vi "XML setApiResponse.vi"(11 "PIM API Response":T1={"#attributes"={"xmlns"="http://www.summitekinstruments.com", "xmlns:xsi"="http://www.w3.org/2001/XMLSchema-instance", "xsi:schemaLocation"="http://www.summitekinstruments.com PIMXMLSchema.xsd"}, "Responses"={"#attributes"={"Legacy"=FALSE}, "Response"=[]}}) -> (3 "Formatted XML":string, 5 "Time to Translate":u32)   [LabVIEW 2011]
uses:
  Controls/PIM.API.RESPONSE.ctl
  Controls/PIM.API.Response.Collection.ctl
  Controls/PIM.API.Response.Unique.ctl
  Controls/PIM.API.Response.Samples.ctl
  WebEngine/LIB/MODULES/TR Module/Triasx.LIB/iQA Sweep Behavior.ctl
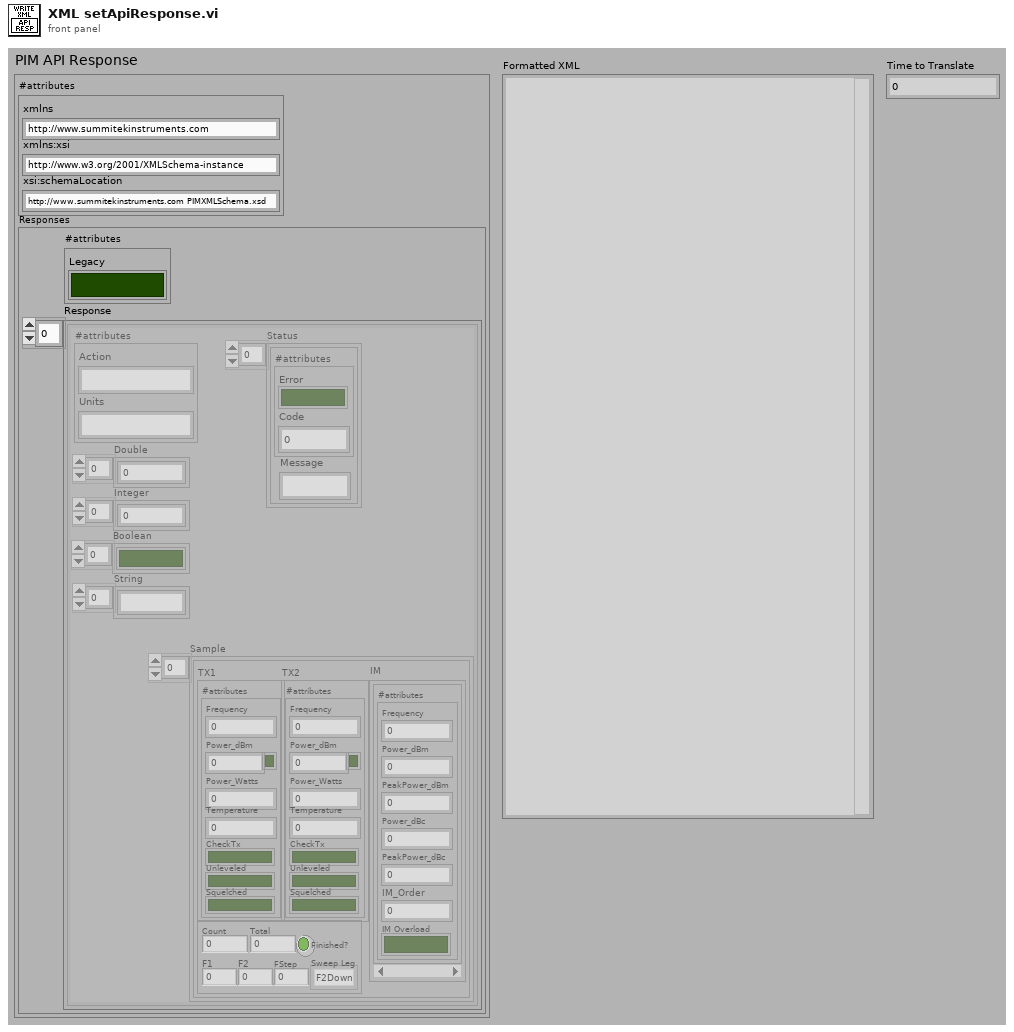
[diagram p1: front panel]
types:
  T1 = typedef "PIM.API.RESPONSE.ctl" = cluster{"#attributes":cluster{"xmlns":string, "xmlns:xsi":string, "xsi:schemaLocation":string}, "Responses":T2}
  T2 = typedef "PIM.API.Response.Collection.ctl" = cluster{"#attributes":cluster{"Legacy":bool}, "Response":T3[]}
  T3 = typedef "PIM.API.Response.Unique.ctl" = cluster{"#attributes":cluster{"Action":string, "Units":string}, "Double":dbl[], "Integer":i32[], "Boolean":bool[], "String":string[], "Sample":T4[], "Status":cluster{"#attributes":cluster{"Error":bool, "Code":i32}, "Message":string}[]}
  T4 = typedef "PIM.API.Response.Samples.ctl" = cluster{"TX1":cluster{"#attributes":cluster{"Frequency":dbl, "Power_dBm":dbl, "Power_Watts":dbl, "CheckTx":bool, "Unleveled":bool, "Squelched":bool, "Temperature":dbl, "ToneOn":bool}}, "TX2":cluster{"#attributes":cluster{"Frequency":dbl, "Power_dBm":dbl, "Power_Watts":dbl, "CheckTx":bool, "Unleveled":bool, "Squelched":bool, "Temperature":dbl, "ToneOn":bool}}, "IM":cluster{"#attributes":cluster{"Frequency":dbl, "Power_dBm":dbl, "PeakPower_dBm":dbl, "Power_dBc":dbl, "PeakPower_dBc":dbl, "IM_Order":u8, "IM Overload":bool}}[], "#attributes":cluster{"Count":u32, "Total":u32, "Finished?":bool, "Sweep Leg":T5, "F1":dbl, "F2":dbl, "FStep":dbl}}
  T5 = typedef "iQA Sweep Behavior.ctl" = enum16{"F2Down", "F1Up", "RxMultiIM"}
  T6 = cluster{"#attributes":cluster{"Error":bool, "Code":i32}, "Message":string}[]
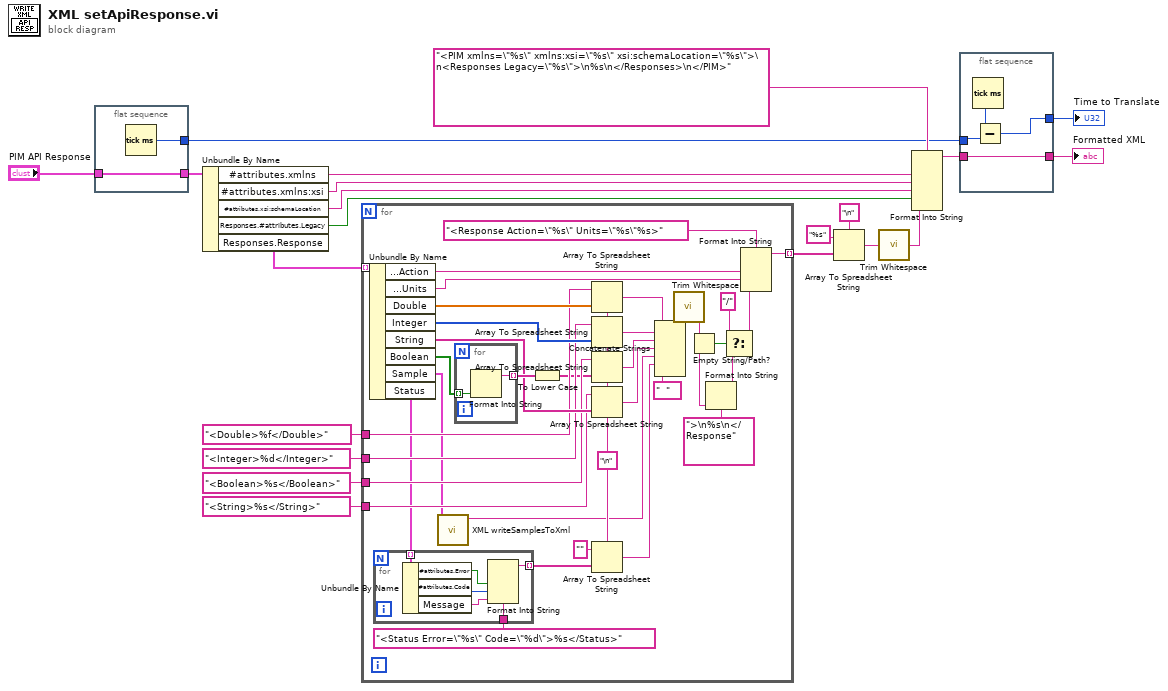
[diagram p0: block diagram]
diagram:
  n1 = flat-sequence {
    tunnel: "PIM API Response" -> [w23]
    tunnel: [w23] -> w6
    tunnel: [w22] -> w3
    frame #0 {
      n2 = Tick Count (ms)() -> (millisecond timer value=w22:u32)
    }
  }
  n3 = Unbundle By Name(w6) -> ("#attributes.xmlns"=w20:string, "#attributes.xmlns:xsi"=w19:string, "#attributes.xsi:schemaLocation"=w18:string, "Responses.#attributes.Legacy"=w17:bool, "Responses.Response"=w16:T3[])
  n4 = for {
    tunnel: w16 -> [w58] mode=indexing
    tunnel: "<Double>%f</Double>" -> [w49]
    tunnel: "<Integer>%d</Integer>" -> [w48]
    tunnel: "<Boolean>%s</Boolean>" -> [w47]
    tunnel: "<String>%s</String>" -> [w46]
    tunnel: [w36] -> w11 mode=indexing
    w42 = "\n" ("delimiter (Tab)")
    n5 = Unbundle By Name(w58) -> ("#attributes.Action"=w56:string, "#attributes.Units"=w55:string, "Double"=w50:dbl[], "Integer"=w51:i32[], "String"=w52:string[], "Boolean"=w54:bool[], "Sample"=w25:T4[], "Status"=w44:T6)
    n6 = for {
      tunnel: [w64] -> w43 mode=indexing
      tunnel: "<Status Error=\"%s\" Code=\"%d\">%s</Status>" -> [w63]
      tunnel: w44 -> [w62] mode=indexing
      n7 = Unbundle By Name(w62) -> ("#attributes.Error"=w61:bool, "#attributes.Code"=w60:i32, "Message"=w59:string)
      n8 = Format Into String(format string=w63, w61, w60, w59) -> (resulting string=w64:string)  [unwired: 2 in, 1 out]
    }
    n9 = call "XML writeSamplesToXml.vi"("Sample"=w25) -> ("Sample XML"=w24:string)  [unwired: 10 in]
    n10 = for {
      tunnel: w54 -> [w66] mode=indexing
      tunnel: [w65] -> w53 mode=indexing
      n11 = Format Into String(w66) -> (resulting string=w65:string)  [unwired: 3 in, 1 out]
    }
    n12 = To Lower Case(string=w53) -> (all lower case string=w26:string[])
    n13 = Array To Spreadsheet String(delimiter (Tab)=w42, array=w50, 3:w49) -> (spreadsheet string=w40:string)
    n14 = Array To Spreadsheet String(delimiter (Tab)=w42, array=w51, 3:w48) -> (spreadsheet string=w38:string)
    n15 = Array To Spreadsheet String(delimiter (Tab)=w42, array=w26, 3:w47) -> (spreadsheet string=w27:string)
    n16 = Array To Spreadsheet String(delimiter (Tab)=w42, array=w52, 3:w46) -> (spreadsheet string=w37:string)
    n17 = Array To Spreadsheet String(delimiter (Tab)=w42, array=w43, 3:"" ("initial string")) -> (spreadsheet string=w39:string)
    n18 = Concatenate Strings(w40, w38, w27, w37, w24, w39, "  " ("initial string")) -> (w41:string)
    n19 = call <vilib>:"Trim Whitespace.vi"("string"=w41) -> ("trimmed string"=w32:string)  [unwired: 1 in]
    n20 = Empty String/Path?(string/path=w32) -> (empty?=w33:bool)
    n21 = Format Into String(format string=">\n%s\n</Response", w32) -> (resulting string=w29:string)  [unwired: 2 in, 1 out]
    n22 = Select(t="/", s=w33, f=w29) -> (s? t:f=w28:string)
    n23 = Format Into String(format string="<Response Action=\"%s\" Units=\"%s\"%s>", w56, w55, w28) -> (resulting string=w36:string)  [unwired: 2 in, 1 out]
  }
  n24 = Array To Spreadsheet String(delimiter (Tab)="\n", array=w11, 3:"%s" ("initial string")) -> (spreadsheet string=w9:string)
  n25 = call <vilib>:"Trim Whitespace.vi"("string"=w9) -> ("trimmed string"=w1:string)  [unwired: 1 in]
  n26 = Format Into String(format string="<PIM xmlns=\"%s\" xmlns:xsi=\"%s\" xsi:schemaLocation=\"%s\">\n<Responses Legacy=\"%s\">\n%s\n</Responses>\n</PIM>", w20, w19, w18, w17, w1) -> (resulting string=w5:string)  [unwired: 2 in, 1 out]
  n27 = flat-sequence {
    tunnel: w5 -> [w70]
    tunnel: [w70] -> w4
    tunnel: w3 -> [w69]
    tunnel: [w67] -> w2
    frame #0 {
      n28 = Tick Count (ms)() -> (millisecond timer value=w68:u32)
      n29 = Subtract(x=w68, y=w69) -> (x-y=w67:u32)
    }
  }
  "Formatted XML" <- w4
  "Time to Translate" <- w2
